vi "Apply Caster Angular Velocity.vi"(8 "error in (no error)":errorcluster, 10 "caster angular velocity":dbl, 11 "caster wheel in":refnum<class "NI_Robotics_Caster Wheel.lvclass">) -> (0 "error out":errorcluster, 3 "caster wheel out":refnum<class "NI_Robotics_Caster Wheel.lvclass">)   [LabVIEW 2017, in "NI_Robotics_Caster Wheel.lvclass"]
uses:
  <vilib>/robotics/Steering/Caster Wheel/NI_Robotics_Caster Wheel.lvclass
  <vilib>/robotics/Steering/Caster Wheel/NI_Robotics_Caster Wheel.lvclass/NI_Robotics_Caster Wheel.ctl
  <vilib>/robotics/Actuation/Motor Communication/Check if Valid.vi
  <vilib>/robotics/Utilities/Generate Error.vi
  <vilib>/robotics/Actuation/Motor Communication/NI_Robotics_Motor Communication.lvclass
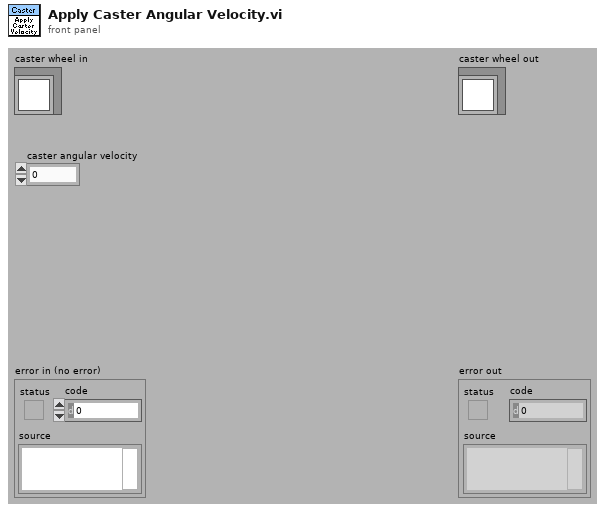
[diagram p1: front panel]
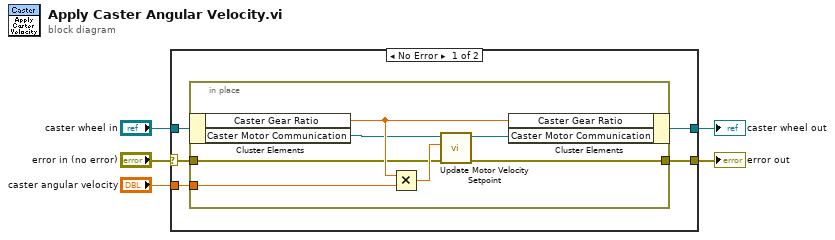
[diagram p0: block diagram]
diagram:
  n1 = case shown="No Error" "error in (no error)" {
    selector: "error in (no error)" -> [w9 w18]
    tunnel: "caster wheel in" -> [w10 w19]
    tunnel: [w8 w19] -> w3
    tunnel: [w7 w18] -> w2
    tunnel: "caster angular velocity" -> [w6 _]
    frame No Error {
      n2 = in-place {
        in-place-border: w9 -> [w12]
        in-place-border: [w11] -> w7
        in-place-border: w6 -> [w16]
        n3 = in-place-cluster #1(w10) -> ("Caster Gear Ratio"=w17:dbl, "Caster Motor Communication"=w14:refnum<class "NI_Robotics_Motor Communication.lvclass">)
        n4 = Multiply(x=w17, y=w16) -> (x*y=w15:dbl)
        n5 = call <vilib>:"Update Motor Velocity Setpoint.vi"("error in (no error)"=w12, "velocity"=w15, "motor communication in"=w14) -> ("error out"=w11:errorcluster, "motor communication out"=w13:refnum<class "NI_Robotics_Motor Communication.lvclass">)  [unwired: 6 in, 1 out]
        n6 = in-place-cluster #1("Caster Gear Ratio"=w17, "Caster Motor Communication"=w13) -> (w8:refnum<class "NI_Robotics_Caster Wheel.lvclass">)
      }
    }
    frame Error {
    }
  }
  "error out" <- w2
  "caster wheel out" <- w3
